vi "NotifyIcon - Set Icon.vi"(8 "error in":errorcluster, 10 "Icon File Path":path=path "C:/myVIs/NotifyIcon/Icons/ni.ico", 11 "NotifyIcon reference in":refnum<k24>) -> (0 "error out":errorcluster, 3 "NotifyIcon reference out":refnum<k24>)   [LabVIEW 2018]
doc: "Sets the Icon shown in the notification area of the Windows task bar."
uses:
  System.Windows.Forms
  System.Drawing
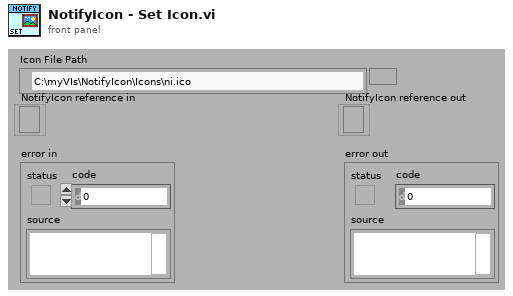
[diagram p1: front panel]
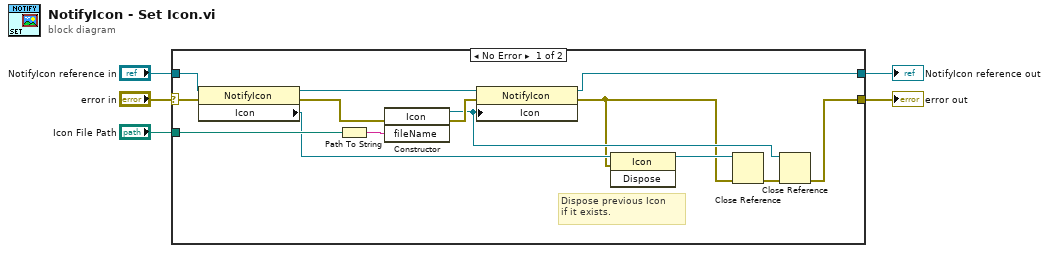
[diagram p0: block diagram]
diagram:
  n1 = case shown="No Error" "error in" {
    selector: "error in" -> [w11 w20]
    tunnel: [w19 w21] -> w5
    tunnel: "Icon File Path" -> [w16 _]
    tunnel: "NotifyIcon reference in" -> [w15 w21]
    tunnel: [w9 w20] -> w2
    frame No Error {
      # "Dispose previous Icon\nif it exists."
      n2 = property class="NotifyIcon"(reference=w15, error in=w11) -> (reference out=w14:refnum<k24>, error out=w13:errorcluster, "Icon"=w12:refnum<k24>)
      n3 = Path To String(path=w16) -> (string=w18:string)
      n4 = constructor class="Icon"(error in=w13, "fileName"=w18) -> (reference out=w7:refnum<k24>, error out=w17:errorcluster)  [unwired: 2 in, 2 out]
      n5 = property class="NotifyIcon"(reference=w14, error in=w17, "Icon"=w7) -> (reference out=w19:refnum<k24>, error out=w6:errorcluster)
      n6 = invoke class="Icon" method="Dispose"(reference=w12, error in=w6) -> (reference out=w10:refnum<k24>)  [unwired: 1 in, 2 out]
      n7 = Close Reference(reference=w10, error in (no error)=w6) -> (error out=w8:errorcluster)
      n8 = Close Reference(reference=w7, error in (no error)=w8) -> (error out=w9:errorcluster)
    }
    frame Error {
    }
  }
  "NotifyIcon reference out" <- w5
  "error out" <- w2
